vi "Save Load Full Setup.vi"(8 "error in (no error)":errorcluster, 9 "Setup Operation (0: Save)":u16(ring) items=["Save", "Load"], 10 "Full Setup File(\"INT:\\full.all\")":string="INT:\\full.all", 11 "VISA resource name":refnum<visa-resource-name>) -> (0 "error out":errorcluster, 3 "VISA resource name out":refnum<visa-resource-name>)   [LabVIEW 2013, in "AWG.lvlib" / "Agilent 3352X Series.lvlib"]
doc: "Recall a complete instrument setup from the named file on the mass storage media so that a user may duplicate instrument conditions from some previous time. \nThe complete instrument setups include: \n(1) Current instrument states which is stored and recalled by Load/Store State.vi\n(2) Names of stored states and ARB Waveforms. \n(3) All other instrument setup information such as LAN and other communications setup, and other user preferences. \n(4) LAN IP address, DHCP status, gateway IP address, hostname, GPIB address \n(5) Number format, beep on/off, display options, and help language"
uses:
  Agilent 3352X Series.lvlib
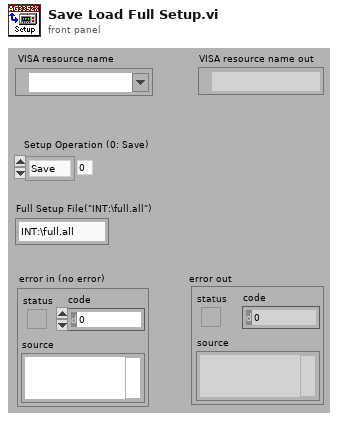
[diagram p1: front panel]
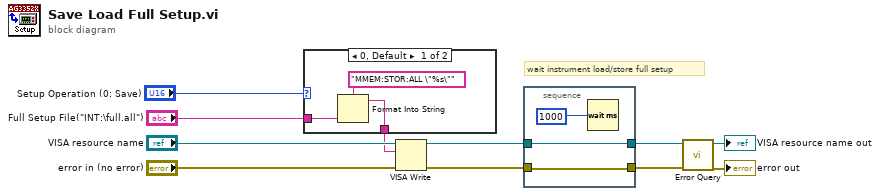
[diagram p0: block diagram]
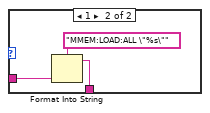
[diagram p2: hidden frame]
diagram:
  # "wait instrument load/store full setup"
  n1 = case shown="0, Default" "Setup Operation (0: Save)" {
    tunnel: "Full Setup File(\"INT:\\full.all\")" -> [w13 w16]
    tunnel: [w12 w15] -> w5
    frame 0, Default {
      n2 = Format Into String(format string="MMEM:STOR:ALL \"%s\"", w13) -> (resulting string=w12:string)  [unwired: 2 in, 1 out]
    }
    frame 1 {
      n3 = Format Into String(format string="MMEM:LOAD:ALL \"%s\"", w16) -> (resulting string=w15:string)  [unwired: 2 in, 1 out]
    }
  }
  n4 = VISA Write(VISA resource name="VISA resource name", write buffer=w5, error in (no error)="error in (no error)") -> (VISA resource name out=w4:refnum<visa-resource-name>, error out=w2:errorcluster)  [unwired: 1 out]
  n5 = stacked-sequence {
    tunnel: w4 -> [w19]
    tunnel: [w19] -> w3
    tunnel: w2 -> [w18]
    tunnel: [w18] -> w1
    frame #0 {
      n6 = Wait (ms)(milliseconds to wait=u32 1000) -> ()  [unwired: 1 out]
    }
  }
  n7 = call "Error Query.vi"("error in (no error)"=w1, "VISA resource name"=w3) -> ("error out"=→"error out":errorcluster, "VISA resource name out"=→"VISA resource name out":refnum<visa-resource-name>)  [unwired: 8 out]
